vi "obj_ClientSrv Server Access State.vi"(0 "method (test access)":T3=enum."test access", 1 "access level":T2=enum."local", 5 "digest":string, 7 "certificate in":string, 9 "LuaVIEW reference {initialize}":T1, 11 "error in (no error)":errorcluster, 12 "access reason":string, 13 "client version":string) -> (8 "certificate out":string, 10 "server name {get name}":string, 15 "error out":errorcluster)   [LabVIEW 2012]
doc: "This server-side object holds the server's access state and provides related methods. The implemented security scheme is described in the manual of the client-server framework. Remotely callable VIs/methods use this object to test the access certificate of the caller. This causes server-side verification that the user of the calling client has been validated at the access level appropriate to the functionality being accessed."
uses:
  typedefs/t_ClientSrv Server Access State Methods.ctl
  typedefs/t_ClientSrv Access Levels.ctl
  luaview/typedefs/t_LuaVIEW Reference.ctl
  luaview/subvis/private/LuaVIEW Pull (flat data).vi
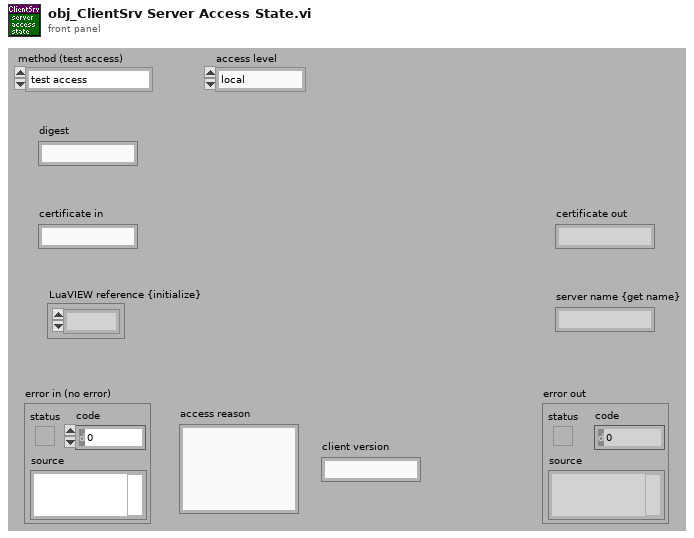
[diagram p1: front panel]
types:
  T1 = typedef "t_LuaVIEW Reference.ctl" = refnum<k1>
  T2 = typedef "t_ClientSrv Access Levels.ctl" = enum16{"observer", "operator", "local"}
  T3 = typedef "t_ClientSrv Server Access State Methods.ctl" = enum16{"initialize", "validate access", "test access", "release access", "get name", "dummy", "cleanup"}
  T4 = cluster{"server name":string, "port number":u32, "access list":string[], "observer password":string, "operator password":string, "access timeout":dbl, "client version":string}
  T5 = cluster{"access":T2, "entropy":dbl, "rand":dbl, "count":dbl}
  T6 = enum32{"invalid app kind", "Development System", "Run Time System", "Student Edition", "Embedded LabVIEW", "Evaluation", "Custom"}
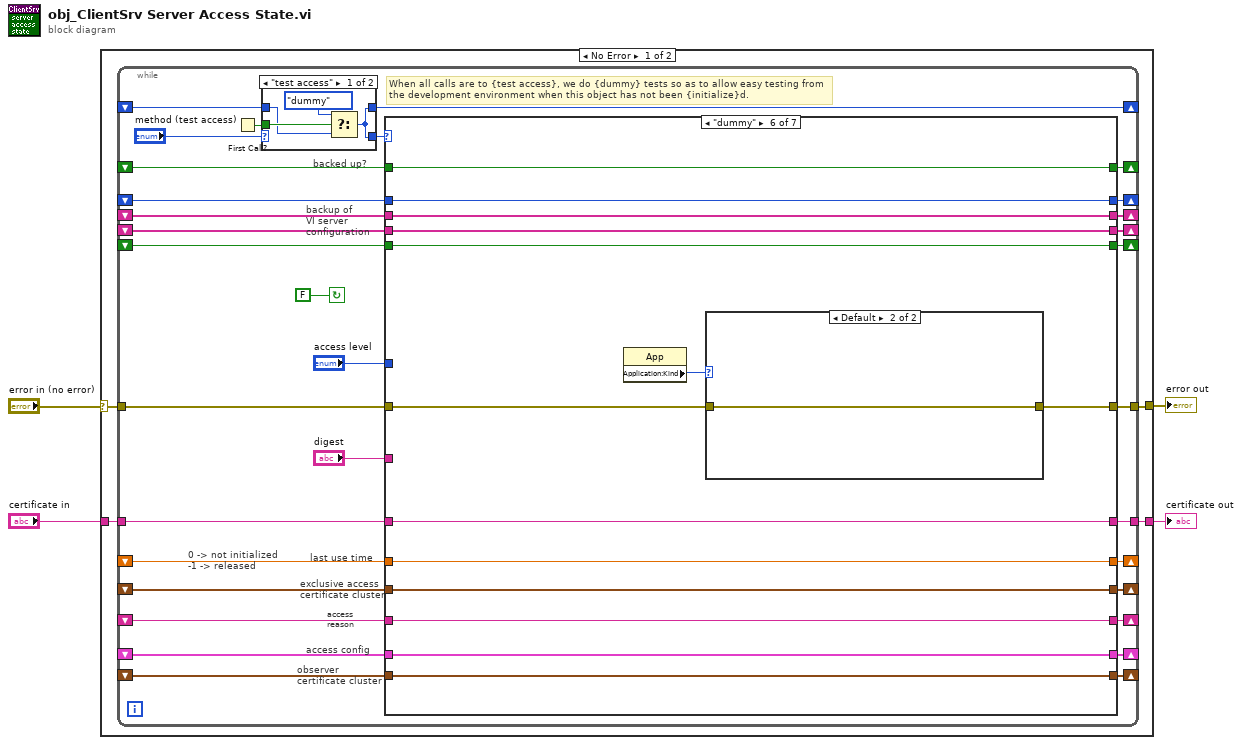
[diagram p0: block diagram]
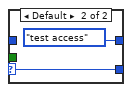
[diagram p2: hidden frame]
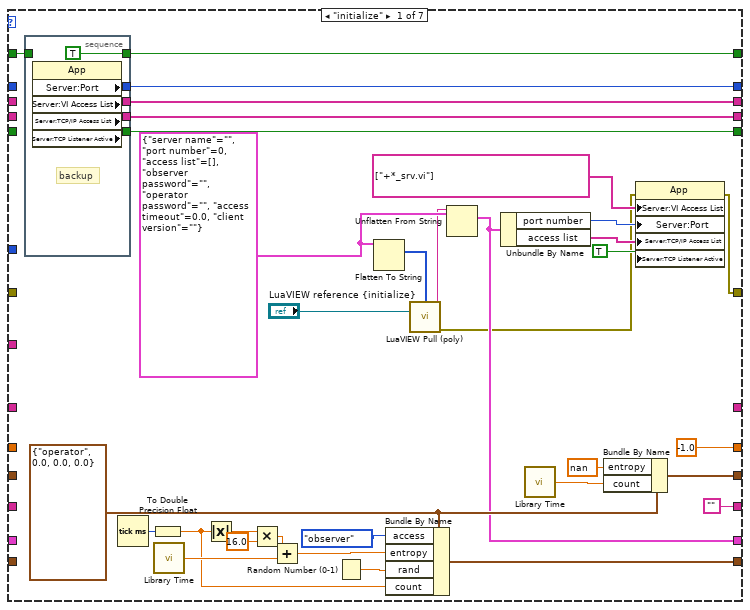
[diagram p3: hidden frame]
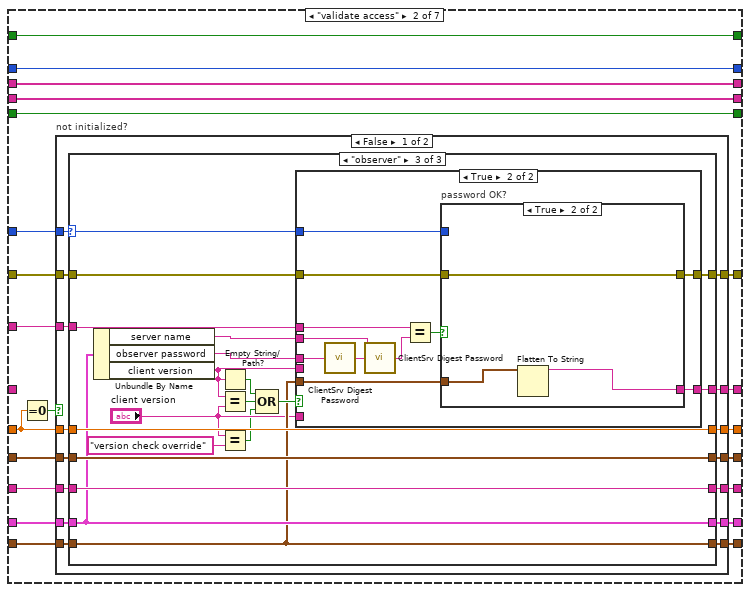
[diagram p4: hidden frame]
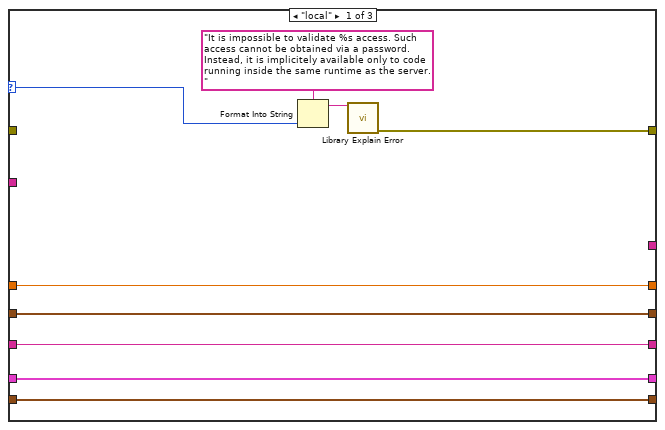
[diagram p5: hidden frame]
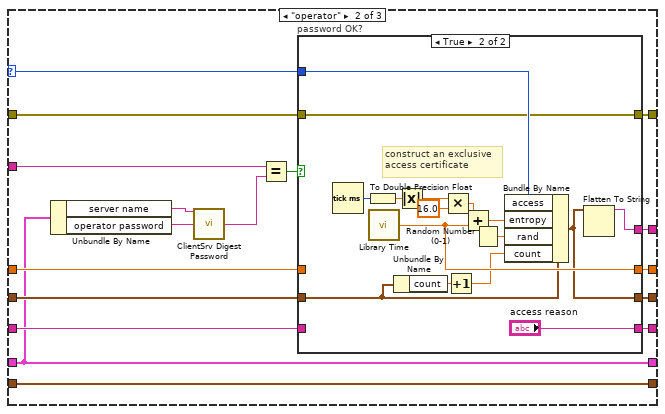
[diagram p6: hidden frame]
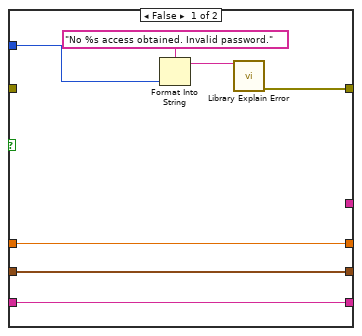
[diagram p7: hidden frame]
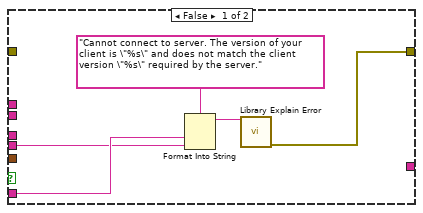
[diagram p8: hidden frame]
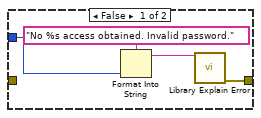
[diagram p9: hidden frame]
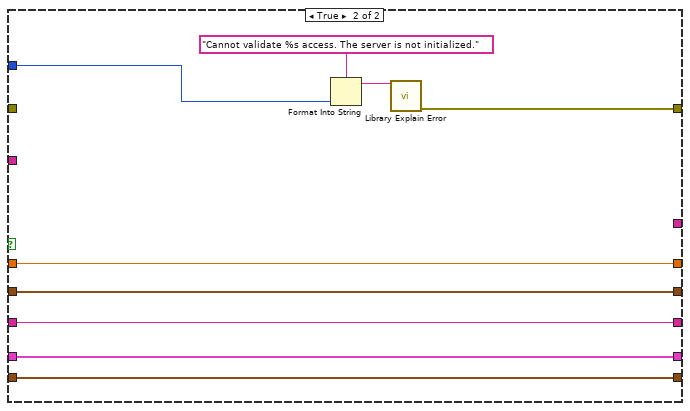
[diagram p10: hidden frame]
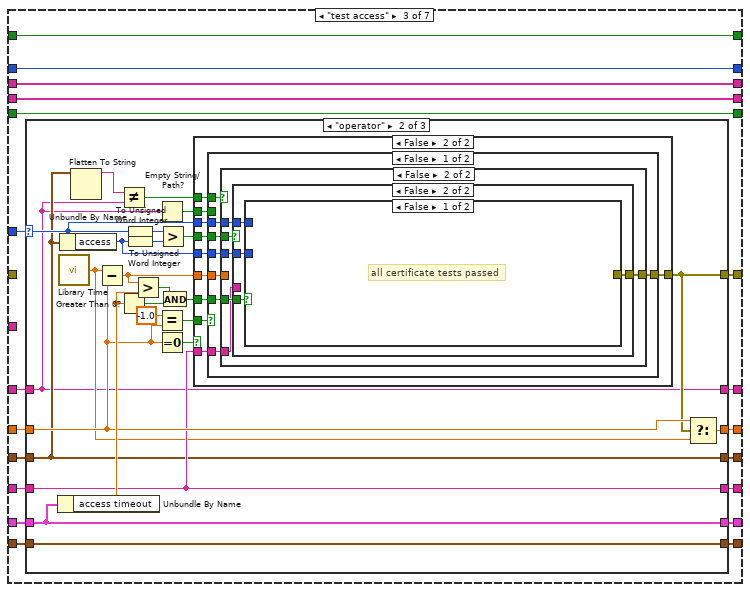
[diagram p11: hidden frame]
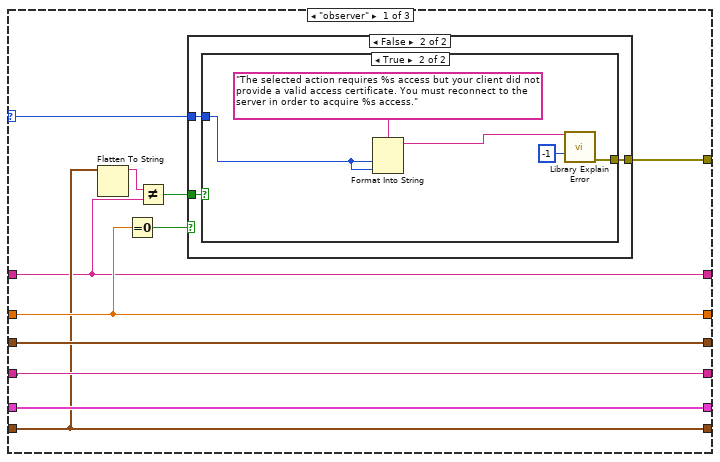
[diagram p12: hidden frame]
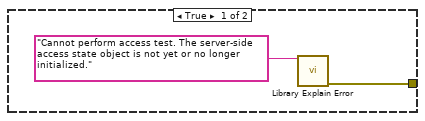
[diagram p13: hidden frame]
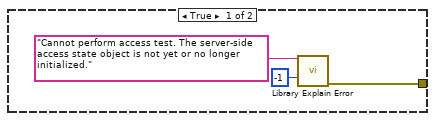
[diagram p15: hidden frame]
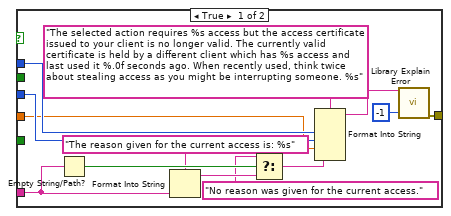
[diagram p16: hidden frame]
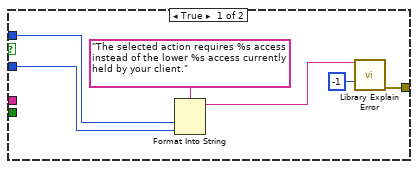
[diagram p17: hidden frame]
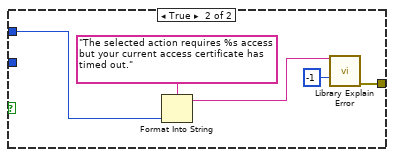
[diagram p18: hidden frame]
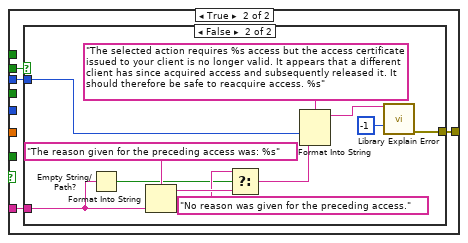
[diagram p19: hidden frame]
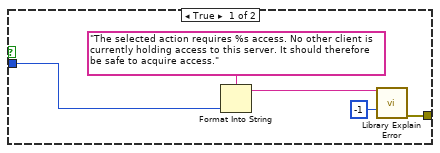
[diagram p20: hidden frame]
diagram:
  n1 = case shown="No Error" "error in (no error)" {
    selector: "error in (no error)" -> [w8 w448]
    tunnel: [w7 w448] -> w3
    tunnel: "certificate in" -> [w6 w447]
    tunnel: [w5 w447] -> w1
    frame No Error {
      n2 = while {
        tunnel: w8 -> [w40]
        tunnel: [w39] -> w7
        shift-right: [w37] -> _
        shift-left: _ -> [w38]
        shift-right: [w31] -> _
        shift-left: _ -> [w30]
        shift-right: [w34] -> _
        shift-left: _ -> [w35]
        shift-right: [w29] -> _
        shift-left: _ -> [w26]
        shift-right: [w28] -> _
        shift-left: _ -> [w25]
        shift-right: [w27] -> _
        shift-left: _ -> [w24]
        shift-right: [w23] -> _
        shift-left: _ -> [w22]
        shift-right: [w20] -> _
        shift-left: _ -> [w21]
        shift-right: [w18] -> _
        shift-left: _ -> [w19]
        shift-right: [w16] -> _
        shift-left: _ -> [w17]
        shift-right: [w14] -> _
        shift-left: _ -> [w12]
        tunnel: w6 -> [w10]
        tunnel: [w9] -> w5
        stop <- FALSE continue-if-true
        # "0 -> not initialized\n-1 -> released"
        # "When all calls are to {test access}, we do {dummy} tests so as to allow easy testing from the development environment when this object has not been {initialize}d."
        # "observer\ncertificate cluster"
        # "access\nreason"
        # "backed up?"
        # "backup of\nVI server\nconfiguration"
        # "last use time"
        # "exclusive access\ncertificate cluster"
        # "access config"
        n3 = First Call?() -> (First Call?: T/F=w13:bool)
        n4 = case shown="\"test access\"" "method (test access)" {
          selector: "method (test access)" -> [_ w45]
          tunnel: [w44 t_ClientSrv_Server_Access_State_Methods."test access" ("method (test access)")] -> w14
          tunnel: [w44 w45] -> w11
          tunnel: w13 -> [w43 _]
          tunnel: w12 -> [w42 _]
          frame "test access" {
            n5 = Select(t=t_ClientSrv_Server_Access_State_Methods."dummy" ("method (test access)"), s=w43, f=w42) -> (s? t:f=w44:T3)
          }
          frame Default {
          }
        }
        n6 = case shown="\"dummy\"" w11 {
          tunnel: w40 -> [_ w99 _ w386 w395 w407 w442]
          tunnel: [w50 w98 w236 w386 w395 w406 w442] -> w39
          tunnel: w38 -> [_ w96 w239 w388 w394 w419 w441]
          tunnel: [w54 w95 w226 w388 w394 w419 w440] -> w37
          tunnel: w30 -> [_ w100 w238 w373 w404 w417 w438]
          tunnel: [w70 w101 w225 w383 w404 w417 w437] -> w31
          tunnel: w35 -> [_ w97 w237 w385 w405 w418 _]
          tunnel: [-1.0 ("seconds since 1Jan1904") w104 w221 w387 w405 w418 0.0 ("seconds since 1Jan1904")] -> w34
          tunnel: "digest" -> [_ w105 _ _ _ _ _]
          tunnel: w10 -> [_ _ w224 w374 w396 w409 _]
          tunnel: [_ w103 w223 w374 w396 w409 _] -> w9
          tunnel: "access level" -> [_ w102 w222 _ _ _ _]
          tunnel: [w76 w91 w235 w379 w403 w416 string[] [] ("Srvr.VIAccessList")] -> w29
          tunnel: [w75 w92 w233 w380 w402 w415 string[] [] ("Srvr.TCPAccessList")] -> w28
          tunnel: [w74 w93 w234 w381 w401 w414 FALSE ("Srvr.TCPActive")] -> w27
          tunnel: w26 -> [_ w91 w235 w379 w403 w416 w434]
          tunnel: w25 -> [_ w92 w233 w380 w402 w415 w433]
          tunnel: w24 -> [_ w93 w234 w381 w401 w414 w432]
          tunnel: [w61 w90 w232 w378 w400 w413 u32 0] -> w23
          tunnel: w22 -> [_ w90 w232 w378 w400 w413 w428]
          tunnel: w21 -> [w73 w89 w231 w377 w399 w412 w426]
          tunnel: [w72 w89 w231 w377 w399 w412 FALSE] -> w20
          tunnel: w19 -> [_ w87 w230 w376 w398 w411 _]
          tunnel: ["" w88 w228 w376 w398 w411 ""] -> w18
          tunnel: w17 -> [_ w86 w229 w375 w397 w410 w423]
          tunnel: [w69 w85 w227 w375 w397 w410 w423] -> w16
          frame "initialize" {
            w57 = T4 {"server name"="", "port number"=0, "access list"=[], "observer password"="", "operator password"="", "access timeout"=0.0, "client version"=""} ("server access config out")
            w68 = T5 {"access"=enum."operator", "entropy"=0.0, "rand"=0.0, "count"=0.0} ("certificate")
            n7 = stacked-sequence {
              tunnel: [w81] -> w76
              tunnel: [w84] -> w75
              tunnel: [w83] -> w74
              tunnel: w73 -> [_]
              tunnel: [TRUE] -> w72
              tunnel: [w80] -> w61
              frame #0 {
                # "backup"
                n8 = property class="App"() -> ("Server:Port"=w80:u32, "Server:VI Access List"=w81:string[], "Server:TCP/IP Access List"=w84:string[], "Server:TCP Listener Active"=w83:bool)  [unwired: 2 in, 2 out]
              }
            }
            n9 = Tick Count (ms)() -> (millisecond timer value=w66:u32)
            n10 = To Double Precision Float(number=w66) -> (double precision float=w48:dbl)
            n11 = call "Library Time.vi"() -> ("time"=w60:dbl)  [unwired: 1 in]
            n12 = Absolute Value(x=w48) -> (abs(x)=w65:dbl)
            n13 = Multiply(x=w65, y=16.0) -> (x*y=w63:dbl)
            n14 = Add(x=w63, y=w60) -> (x+y=w62:dbl)
            n15 = Random Number (0-1)() -> (number: 0 to 1=w47:dbl)
            n16 = Flatten To String(anything=w57) -> (type string=w58:i16[])  [unwired: 3 in, 2 out]
            n17 = Bundle By Name(cluster=w68, "access"=t_ClientSrv_Access_Levels."observer", "entropy"=w62, "rand"=w47, "count"=w48) -> (w69:T5)
            n18 = call-poly "LuaVIEW Pull (poly).vi"("type descriptor"=w58, "LuaVIEW reference in"="LuaVIEW reference {initialize}") -> ("flat data"=w56:string, "error out"=w51:errorcluster)  [unwired: 11 in, 1 out]
            n19 = Unflatten From String(type=w57, binary string=w56) -> (value=w54:T4)  [unwired: 3 in, 2 out]
            n20 = Unbundle By Name(w54) -> ("port number"=w53:u32, "access list"=w52:string[])
            n21 = call "Library Time.vi"() -> ("time"=w59:dbl)  [unwired: 1 in]
            n22 = Bundle By Name(cluster=w68, "entropy"=nan, "count"=w59) -> (w70:T5)
            n23 = property class="App"(error in=w51, "Server:VI Access List"=string[] ["+*_srv.vi"], "Server:Port"=w53, "Server:TCP/IP Access List"=w52, "Server:TCP Listener Active"=TRUE) -> (error out=w50:errorcluster)  [unwired: 1 in, 1 out]
          }
          frame "validate access" {
            n24 = Equal To 0?(x=w97) -> (x = 0?=w94:bool)
            n25 = case "not initialized?" shown="False" w94 {
              tunnel: w105 -> [w108 _]
              tunnel: [w120 w214] -> w104
              tunnel: w96 -> [w107 w216]
              tunnel: [w119 _] -> w103
              tunnel: w102 -> [w106 w217]
              tunnel: [w118 w215] -> w101
              tunnel: w100 -> [w117 w215]
              tunnel: w99 -> [w116 _]
              tunnel: [w115 w220] -> w98
              tunnel: w97 -> [w114 w214]
              tunnel: [w111 w216] -> w95
              tunnel: [w113 w213] -> w88
              tunnel: w87 -> [w112 w213]
              tunnel: w86 -> [w110 w212]
              tunnel: [w109 w212] -> w85
              frame False {
                n26 = case shown="\"observer\"" w106 {
                  selector: w106 -> [w127 w134 w184]
                  tunnel: [w125 w146 w181] -> w120
                  tunnel: [_ w145 w188] -> w119
                  tunnel: [w124 w144 w180] -> w118
                  tunnel: w117 -> [w124 w143 w180]
                  tunnel: w116 -> [_ w142 w187]
                  tunnel: [w126 w141 w186] -> w115
                  tunnel: w114 -> [w125 w140 w181]
                  tunnel: [w123 w138 w179] -> w113
                  tunnel: w112 -> [w123 w137 w179]
                  tunnel: [w122 w131 w178] -> w111
                  tunnel: w110 -> [w121 w130 w174]
                  tunnel: [w121 w130 w174] -> w109
                  tunnel: w108 -> [_ w136 w185]
                  tunnel: w107 -> [w122 w131 w178]
                  frame "local" {
                    n27 = Format Into String(format string="It is impossible to validate %s access. Such access cannot be obtained via a password. Instead, it is implicitely available only to code running inside the same runtime as the server." ("explanation"), w127) -> (resulting string=w128:string)  [unwired: 2 in, 1 out]
                    n28 = call "Library Explain Error.vi"("explanation prefix (none)"=w128) -> ("explained error"=w126:errorcluster)  [unwired: 14 in]
                  }
                  frame "operator" {
                    n29 = Unbundle By Name(w131) -> ("server name"=w132:string, "operator password"=w133:string)
                    n30 = call "ClientSrv Digest Password.vi"("server name (none)"=w132, "password"=w133) -> ("SHA-1 digest"=w135:string)  [unwired: 13 in]
                    n31 = Equal?(x=w136, y=w135) -> (x = y?=w139:bool)
                    n32 = case "password OK?" shown="True" w139 {
                      tunnel: [_ w168] -> w145
                      tunnel: [w153 w169] -> w146
                      tunnel: w134 -> [w149 w164]
                      tunnel: w140 -> [w153 _]
                      tunnel: [w152 w166] -> w144
                      tunnel: w143 -> [w152 w167]
                      tunnel: w142 -> [_ w163]
                      tunnel: [w151 w163] -> w141
                      tunnel: [w147 "access reason"] -> w138
                      tunnel: w137 -> [w147 _]
                      frame False {
                        n33 = Format Into String(format string="No %s access obtained. Invalid password." ("explanation"), w149) -> (resulting string=w148:string)  [unwired: 2 in, 1 out]
                        n34 = call "Library Explain Error.vi"("explanation prefix (none)"=w148) -> ("explained error"=w151:errorcluster)  [unwired: 14 in]
                      }
                      frame True {
                        # "construct an exclusive\naccess certificate"
                        n35 = Tick Count (ms)() -> (millisecond timer value=w162:u32)
                        n36 = To Double Precision Float(number=w162) -> (double precision float=w161:dbl)
                        n37 = call "Library Time.vi"() -> ("time"=w169:dbl)  [unwired: 1 in]
                        n38 = Unbundle By Name(w167) -> ("count"=w156:dbl)
                        n39 = Absolute Value(x=w161) -> (abs(x)=w160:dbl)
                        n40 = Multiply(x=w160, y=16.0) -> (x*y=w158:dbl)
                        n41 = Increment(x=w156) -> (x+1=w155:dbl)
                        n42 = Add(x=w158, y=w169) -> (x+y=w157:dbl)
                        n43 = Random Number (0-1)() -> (number: 0 to 1=w154:dbl)
                        n44 = Bundle By Name(cluster=w167, "access"=w164, "entropy"=w157, "rand"=w154, "count"=w155) -> (w166:T5)
                        n45 = Flatten To String(anything=w166) -> (data string=w168:string)  [unwired: 3 in, 2 out]
                      }
                    }
                  }
                  frame "observer" {
                    n46 = Unbundle By Name(w178) -> ("server name"=w183:string, "observer password"=w182:string, "client version"=w173:string)
                    n47 = Empty String/Path?(string/path=w173) -> (empty?=w177:bool)
                    n48 = Equal?(x=w173, y="client version") -> (x = y?=w176:bool)
                    n49 = Equal?(x="client version", y="version check override") -> (x = y?=w171:bool)
                    n50 = Compound Arithmetic op=OR(w177, w176, w171) -> (w175:bool)
                    n51 = case shown="True" w175 {
                      tunnel: [_ w204] -> w188
                      tunnel: w187 -> [_ w203]
                      tunnel: [w189 w202] -> w186
                      tunnel: w185 -> [_ w200]
                      tunnel: w184 -> [_ w198]
                      tunnel: w183 -> [_ w197]
                      tunnel: w182 -> [_ w195]
                      tunnel: w174 -> [_ w194]
                      tunnel: w173 -> [w190 _]
                      tunnel: "client version" -> [w191 _]
                      frame False {
                        n52 = Format Into String(format string="Cannot connect to server. The version of your client is \"%s\" and does not match the client version \"%s\" required by the server.", w191, w190) -> (resulting string=w193:string)  [unwired: 2 in, 1 out]
                        n53 = call "Library Explain Error.vi"("explanation prefix (none)"=w193) -> ("explained error"=w189:errorcluster)  [unwired: 14 in]
                      }
                      frame True {
                        n54 = call "ClientSrv Digest Password.vi"("password"=w195) -> ("SHA-1 digest"=w196:string)  [unwired: 14 in]
                        n55 = call "ClientSrv Digest Password.vi"("server name (none)"=w197, "password"=w196) -> ("SHA-1 digest"=w199:string)  [unwired: 13 in]
                        n56 = Equal?(x=w200, y=w199) -> (x = y?=w201:bool)
                        n57 = case "password OK?" shown="True" w201 {
                          tunnel: [_ w211] -> w204
                          tunnel: w198 -> [w206 _]
                          tunnel: w203 -> [_ w210]
                          tunnel: [w208 w210] -> w202
                          tunnel: w194 -> [_ w209]
                          frame False {
                            n58 = Format Into String(format string="No %s access obtained. Invalid password." ("explanation"), w206) -> (resulting string=w205:string)  [unwired: 2 in, 1 out]
                            n59 = call "Library Explain Error.vi"("explanation prefix (none)"=w205) -> ("explained error"=w208:errorcluster)  [unwired: 14 in]
                          }
                          frame True {
                            n60 = Flatten To String(anything=w209) -> (data string=w211:string)  [unwired: 3 in, 2 out]
                          }
                        }
                      }
                    }
                  }
                }
              }
              frame True {
                n61 = Format Into String(format string="Cannot validate %s access. The server is not initialized." ("explanation"), w217) -> (resulting string=w219:string)  [unwired: 2 in, 1 out]
                n62 = call "Library Explain Error.vi"("explanation prefix (none)"=w219) -> ("explained error"=w220:errorcluster)  [unwired: 14 in]
              }
            }
          }
          frame "test access" {
            n63 = case shown="\"operator\"" w222 {
              selector: w222 -> [w243 w265 w363]
              tunnel: w239 -> [w249 w267 w370]
              tunnel: w238 -> [w246 w263 w369]
              tunnel: w237 -> [w247 w274 w366]
              tunnel: [w245 w271 w362] -> w236
              tunnel: w224 -> [w240 w261 w367]
              tunnel: w230 -> [w250 w266 w371]
              tunnel: w229 -> [w242 w268 w368]
              tunnel: [w250 w266 w371] -> w228
              tunnel: [w242 w268 w368] -> w227
              tunnel: [w249 w267 w370] -> w226
              tunnel: [w246 w263 w369] -> w225
              tunnel: [w240 w261 w367] -> w223
              tunnel: [w247 w283 w366] -> w221
              frame "observer" {
                n64 = Flatten To String(anything=w242) -> (data string=w241:string)  [unwired: 3 in, 2 out]
                n65 = Equal To 0?(x=w247) -> (x = 0?=w248:bool)
                n66 = Not Equal?(x=w241, y=w240) -> (x != y?=w244:bool)
                n67 = case shown="False" w248 {
                  tunnel: [w252 w255] -> w245
                  tunnel: w244 -> [_ w254]
                  tunnel: w243 -> [_ w253]
                  frame True {
                    n68 = call "Library Explain Error.vi"("explanation prefix (none)"="Cannot perform access test. The server-side access state object is not yet or no longer initialized." ("explanation")) -> ("explained error"=w252:errorcluster)  [unwired: 14 in]
                  }
                  frame False {
                    n69 = case shown="True" w254 {
                      tunnel: [_ w260] -> w255
                      tunnel: w253 -> [_ w257]
                      frame False {
                      }
                      frame True {
                        n70 = Format Into String(format string="The selected action requires %s access but your client did not provide a valid access certificate. You must reconnect to the server in order to acquire %s access." ("explanation"), w257, w257) -> (resulting string=w258:string)  [unwired: 2 in, 1 out]
                        n71 = call "Library Explain Error.vi"("explanation prefix (none)"=w258, "skip levels (0)"=-1) -> ("explained error"=w260:errorcluster)  [unwired: 13 in]
                      }
                    }
                  }
                }
              }
              frame "operator" {
                n72 = Unbundle By Name(w267) -> ("access timeout"=w285:dbl)
                n73 = call "Library Time.vi"() -> ("time"=w264:dbl)  [unwired: 1 in]
                n74 = Unbundle By Name(w263) -> ("access"=w277:T2)
                n75 = Flatten To String(anything=w263) -> (data string=w262:string)  [unwired: 3 in, 2 out]
                n76 = Subtract(x=w264, y=w274) -> (x-y=w276:dbl)
                n77 = Not Equal?(x=w262, y=w261) -> (x != y?=w279:bool)
                n78 = Greater Than 0?(x=w285) -> (x > 0?=w275:bool)
                n79 = To Unsigned Word Integer(number=w265) -> (unsigned 16bit integer=w282:u16)
                n80 = To Unsigned Word Integer(number=w277) -> (unsigned 16bit integer=w281:u16)
                n81 = Greater?(x=w276, y=w285) -> (0:w284:bool)
                n82 = Empty String/Path?(string/path=w261) -> (empty?=w269:bool)
                n83 = Equal?(x=-1.0, y=w274) -> (x = y?=w272:bool)
                n84 = Equal To 0?(x=w274) -> (x = 0?=w280:bool)
                n85 = Greater?(x=w282, y=w281) -> (0:w278:bool)
                n86 = And(x=w284, y=w275) -> (x .and. y?=w270:bool)
                n87 = case shown="False" w280 {
                  tunnel: [w288 w298] -> w271
                  tunnel: w279 -> [_ w297]
                  tunnel: w265 -> [_ w296]
                  tunnel: w276 -> [_ w295]
                  tunnel: w278 -> [_ w294]
                  tunnel: w277 -> [_ w293]
                  tunnel: w272 -> [_ w292]
                  tunnel: w270 -> [_ w291]
                  tunnel: w269 -> [_ w290]
                  tunnel: w266 -> [_ w289]
                  frame True {
                    n88 = call "Library Explain Error.vi"("explanation prefix (none)"="Cannot perform access test. The server-side access state object is not yet or no longer initialized." ("explanation"), "skip levels (0)"=-1) -> ("explained error"=w288:errorcluster)  [unwired: 13 in]
                  }
                  frame False {
                    n89 = case shown="False" w292 {
                      tunnel: [w306 w344] -> w298
                      tunnel: w297 -> [w305 _]
                      tunnel: w296 -> [w304 w343]
                      tunnel: w295 -> [w303 _]
                      tunnel: w294 -> [w302 _]
                      tunnel: w293 -> [w301 _]
                      tunnel: w291 -> [w300 _]
                      tunnel: w290 -> [_ w342]
                      tunnel: w289 -> [w299 w341]
                      frame False {
                        n90 = case shown="False" w305 {
                          tunnel: [w319 w325] -> w306
                          tunnel: w304 -> [w315 w322]
                          tunnel: w303 -> [w314 _]
                          tunnel: w302 -> [_ w324]
                          tunnel: w301 -> [w316 w323]
                          tunnel: w300 -> [_ w321]
                          tunnel: w299 -> [w312 w320]
                          frame True {
                            n91 = Empty String/Path?(string/path=w312) -> (empty?=w313:bool)
                            n92 = Format Into String(format string="The reason given for the current access is: %s", w312) -> (resulting string=w310:string)  [unwired: 2 in, 1 out]
                            n93 = Select(t="No reason was given for the current access.", s=w313, f=w310) -> (s? t:f=w308:string)
                            n94 = Format Into String(format string="The selected action requires %s access but the access certificate issued to your client is no longer valid. The currently valid certificate is held by a different client which has %s access and last used it %.0f seconds ago. When recently used, think twice about stealing access as you might be interrupting someone. %s" ("explanation"), w315, w316, w314, w308) -> (resulting string=w317:string)  [unwired: 2 in, 1 out]
                            n95 = call "Library Explain Error.vi"("explanation prefix (none)"=w317, "skip levels (0)"=-1) -> ("explained error"=w319:errorcluster)  [unwired: 13 in]
                          }
                          frame False {
                            n96 = case shown="False" w324 {
                              tunnel: [w331 w335] -> w325
                              tunnel: w323 -> [w327 w333]
                              tunnel: w322 -> [w328 w334]
                              tunnel: w321 -> [_ w332]
                              tunnel: w320 -> [_ _]
                              frame True {
                                n97 = Format Into String(format string="The selected action requires %s access instead of the lower %s access currently held by your client." ("explanation"), w328, w327) -> (resulting string=w329:string)  [unwired: 2 in, 1 out]
                                n98 = call "Library Explain Error.vi"("explanation prefix (none)"=w329, "skip levels (0)"=-1) -> ("explained error"=w331:errorcluster)  [unwired: 13 in]
                              }
                              frame False {
                                n99 = case shown="False" w332 {
                                tunnel: [_ w340] -> w335
                                tunnel: w334 -> [_ w337]
                                tunnel: w333 -> [_ _]
                                frame False {
                                # "all certificate tests passed"
                                }
                                frame True {
                                n100 = Format Into String(format string="The selected action requires %s access but your current access certificate has timed out." ("explanation"), w337) -> (resulting string=w338:string)  [unwired: 2 in, 1 out]
                                n101 = call "Library Explain Error.vi"("explanation prefix (none)"=w338, "skip levels (0)"=-1) -> ("explained error"=w340:errorcluster)  [unwired: 13 in]
                                }
                                }
                              }
                            }
                          }
                        }
                      }
                      frame True {
                        n102 = case shown="False" w342 {
                          tunnel: [w349 w360] -> w344
                          tunnel: w343 -> [w346 w357]
                          tunnel: w341 -> [_ w352]
                          frame True {
                            n103 = Format Into String(format string="The selected action requires %s access. No other client is currently holding access to this server. It should therefore be safe to acquire access." ("explanation"), w346) -> (resulting string=w347:string)  [unwired: 2 in, 1 out]
                            n104 = call "Library Explain Error.vi"("explanation prefix (none)"=w347, "skip levels (0)"=-1) -> ("explained error"=w349:errorcluster)  [unwired: 13 in]
                          }
                          frame False {
                            n105 = Empty String/Path?(string/path=w352) -> (empty?=w353:bool)
                            n106 = Format Into String(format string="The reason given for the preceding access was: %s", w352) -> (resulting string=w355:string)  [unwired: 2 in, 1 out]
                            n107 = Select(t="No reason was given for the preceding access.", s=w353, f=w355) -> (s? t:f=w351:string)
                            n108 = Format Into String(format string="The selected action requires %s access but the access certificate issued to your client is no longer valid. It appears that a different client has since acquired access and subsequently released it. It should therefore be safe to reacquire access. %s" ("explanation"), w357, w351) -> (resulting string=w358:string)  [unwired: 2 in, 1 out]
                            n109 = call "Library Explain Error.vi"("explanation prefix (none)"=w358, "skip levels (0)"=-1) -> ("explained error"=w360:errorcluster)  [unwired: 13 in]
                          }
                        }
                      }
                    }
                  }
                }
                n110 = Select(t=w274, s=w271, f=w264) -> (s? t:f=w283:dbl)
              }
              frame "local" {
                n111 = Format Into String(format string="The called VI/method requires %s access and is not available for remote calling. Such access is implicitely available only to code running inside the same runtime as the server." ("explanation"), w363) -> (resulting string=w364:string)  [unwired: 2 in, 1 out]
                n112 = call "Library Explain Error.vi"("explanation prefix (none)"=w364, "skip levels (0)"=1) -> ("explained error"=w362:errorcluster)  [unwired: 13 in]
              }
            }
          }
          frame "release access" {
            n113 = Flatten To String(anything=w373) -> (data string=w372:string)  [unwired: 3 in, 2 out]
            n114 = Equal?(x=w372, y=w374) -> (x = y?=w382:bool)
            n115 = Select(t=-1.0, s=w382, f=w385) -> (s? t:f=w387:dbl)
            n116 = case shown="True" w382 {
              tunnel: w373 -> [w389 w391]
              tunnel: [w389 w390] -> w383
              frame False {
              }
              frame True {
                n117 = Bundle By Name(cluster=w391, "entropy"=nan) -> (w390:T5)
              }
            }
          }
          frame "get name" {
            n118 = Unbundle By Name(w394) -> ("server name"=→"server name {get name}":string)
          }
          frame "dummy" {
            n119 = property class="App"() -> ("Application:Kind"=w408:T6)  [unwired: 2 in, 2 out]
            n120 = case shown="Default" w408 {
              tunnel: w407 -> [_ w422]
              tunnel: [w421 w422] -> w406
              frame "Run Time System" {
                n121 = call "Library Explain Error.vi"("explanation prefix (none)"="Dummy access tests, which occur when this object is never initialized or otherwise called with methods other than {test access}, are allowed only when running under the LabVIEW development environment.") -> ("explained error"=w421:errorcluster)  [unwired: 14 in]
              }
              frame Default {
              }
            }
          }
          frame "cleanup" {
            w439 = "safhgjgt#$dkcierfiueouh"
            n122 = case shown="True" w426 {
              tunnel: w434 -> [_ w444]
              tunnel: w433 -> [_ w446]
              tunnel: w432 -> [_ w445]
              tunnel: w428 -> [_ w443]
              frame False {
              }
              frame True {
                # "restore"
                n123 = property class="App"("Server:Port"=w443, "Server:VI Access List"=w444, "Server:TCP/IP Access List"=w446, "Server:TCP Listener Active"=w445) -> ()  [unwired: 2 in, 2 out]
              }
            }
            n124 = Bundle By Name(cluster=w441, "observer password"=w439, "operator password"=w439) -> (w440:T4)
            n125 = Bundle By Name(cluster=w438, "entropy"=nan) -> (w437:T5)
          }
        }
      }
    }
    frame Error {
    }
  }
  "error out" <- w3
  "certificate out" <- w1
